vi "TEMPLATE_Constructor.vi"(8 "Error In":errorcluster) -> (0 "Error Out":errorcluster, 3 "%TYPE% Out":refnum<class "LQSerialData.lvclass">)   [LabVIEW 2013, in "Template.lvlib" / "LQSerialData.lvclass"]
uses:
  LQSerialData.lvclass
  LQSerialData.lvclass/LQSerialData.ctl
  Template.lvlib
  LQWidgetEngine/LQWidgetEngine.lvclass
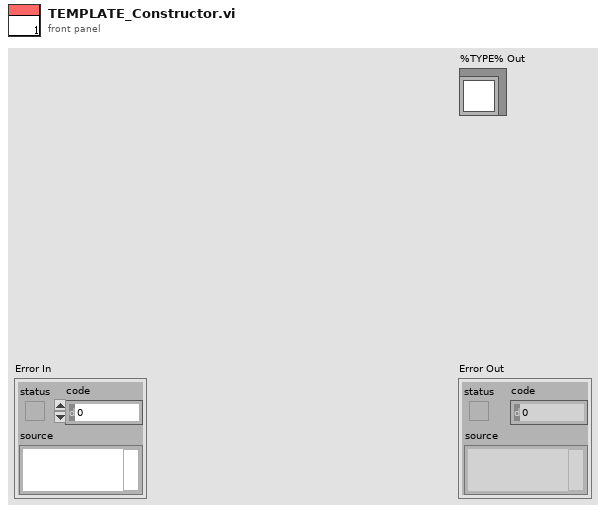
[diagram p1: front panel]
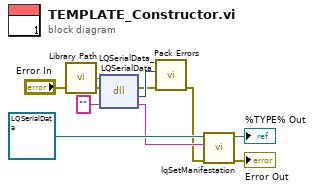
[diagram p0: block diagram]
diagram:
  n1 = call "Library Path.vi"() -> ("Library Path"=w5:path)
  n2 = dll-call lib="?" fn="LQSerialData_LQSerialData"(path in=w5, error in="Error In", "_instance"="") -> (error out=w3:errorcluster, "errorCode"=w4:i32, "_instance"=w6:string)  [unwired: 1 in, 1 out]
  n3 = call "Pack Errors.vi"("Error In"=w3, "Error Code"=w4) -> ("Error Out"=w2:errorcluster)  [unwired: 9 in]
  n4 = call "lqSetManifestation.vi"("Error In"=w2, "Manifestation"=w6, "LQSerialData in"=refnum<class "LQSerialData.lvclass"> refnum ("%TYPE%")) -> ("Error Out"=→"Error Out":errorcluster, "LQSerialData out"=→"%TYPE% Out":refnum<class "LQSerialData.lvclass">)  [unwired: 7 in]
